vi "FontToObject.vi"(5 "FontName":string, 7 "emSize":sgl, 9 "style":i32(ring) items=["Regular"=0, "Bold"=1, "Italic"=2, "Underline"=4, "Strikeout"=8], 11 "error in (no error)":errorcluster) -> (6 "FontObject":refnum<k24>, 15 "error out":errorcluster)   [LabVIEW 2018, in "DataGridView.lvclass"]
doc: "Converts a font name and size to a System.Drawing.Font object"
uses:
  DataGridView.lvclass
  System.Drawing
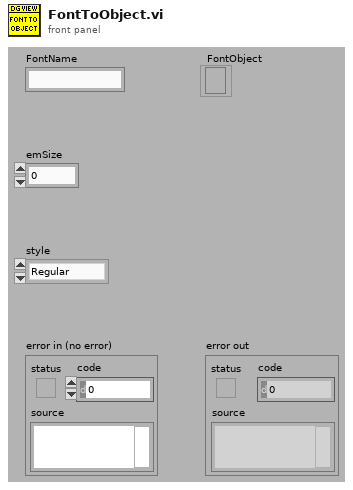
[diagram p1: front panel]
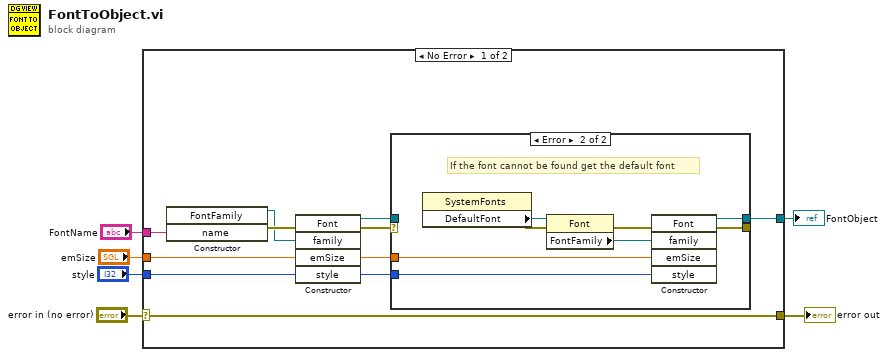
[diagram p0: block diagram]
diagram:
  n1 = case shown="No Error" "error in (no error)" {
    selector: "error in (no error)" -> [w15 w26]
    tunnel: [w15 w26] -> w5
    tunnel: "FontName" -> [w10 _]
    tunnel: "emSize" -> [w9 _]
    tunnel: [w8 _] -> w2
    tunnel: "style" -> [w7 _]
    frame No Error {
      n2 = constructor class="FontFamily"("name"=w10) -> (reference out=w13:refnum<k24>, error out=w14:errorcluster)  [unwired: 3 in, 2 out]
      n3 = constructor class="Font"(error in=w14, "family"=w13, "emSize"=w9, "style"=w7) -> (reference out=w11:refnum<k24>, error out=w12:errorcluster)  [unwired: 2 in, 4 out]
      n4 = case shown="Error" w12 {
        selector: w12 -> [w17 _]
        tunnel: [w17 w22] -> _
        tunnel: w11 -> [w16 _]
        tunnel: [w16 w20] -> w8
        tunnel: w9 -> [_ w19]
        tunnel: w7 -> [_ w18]
        frame No Error {
        }
        frame Error {
          # "If the font cannot be found get the default font"
          n5 = property class="SystemFonts"() -> (error out=w24:errorcluster, "DefaultFont"=w25:refnum<k24>)  [unwired: 2 in, 1 out]
          n6 = property class="Font"(reference=w25, error in=w24) -> (error out=w23:errorcluster, "FontFamily"=w21:refnum<k24>)  [unwired: 1 out]
          n7 = constructor class="Font"(error in=w23, "family"=w21, "emSize"=w19, "style"=w18) -> (reference out=w20:refnum<k24>, error out=w22:errorcluster)  [unwired: 2 in, 4 out]
        }
      }
    }
    frame Error {
    }
  }
  "error out" <- w5
  "FontObject" <- w2
